vi "ServoSet.vi"(8 "error in":errorcluster, 10 "manual":dbl=0.03, 11 "Radio Buttons":T1(radio)) -> (0 "error out":errorcluster)   [LabVIEW 2016]
uses:
  <vilib>/DAQmx/create/channels.llb/DAQmx Create Channel (CO-Pulse Generation-Frequency).vi
  <vilib>/DAQmx/configure/timing.llb/DAQmx Timing (Implicit).vi
panel:
  in  "new duty cycle 2":dbl=0.5 min=0.001 max=0.999 step=0.001 format="%.6f"
  in  "idle state":i32(ring)=10214 items=["High"=10192, "Low"=10214]
  # "input roughly 0.008 ... 0.045"
  # "1\n24\n37\n48"
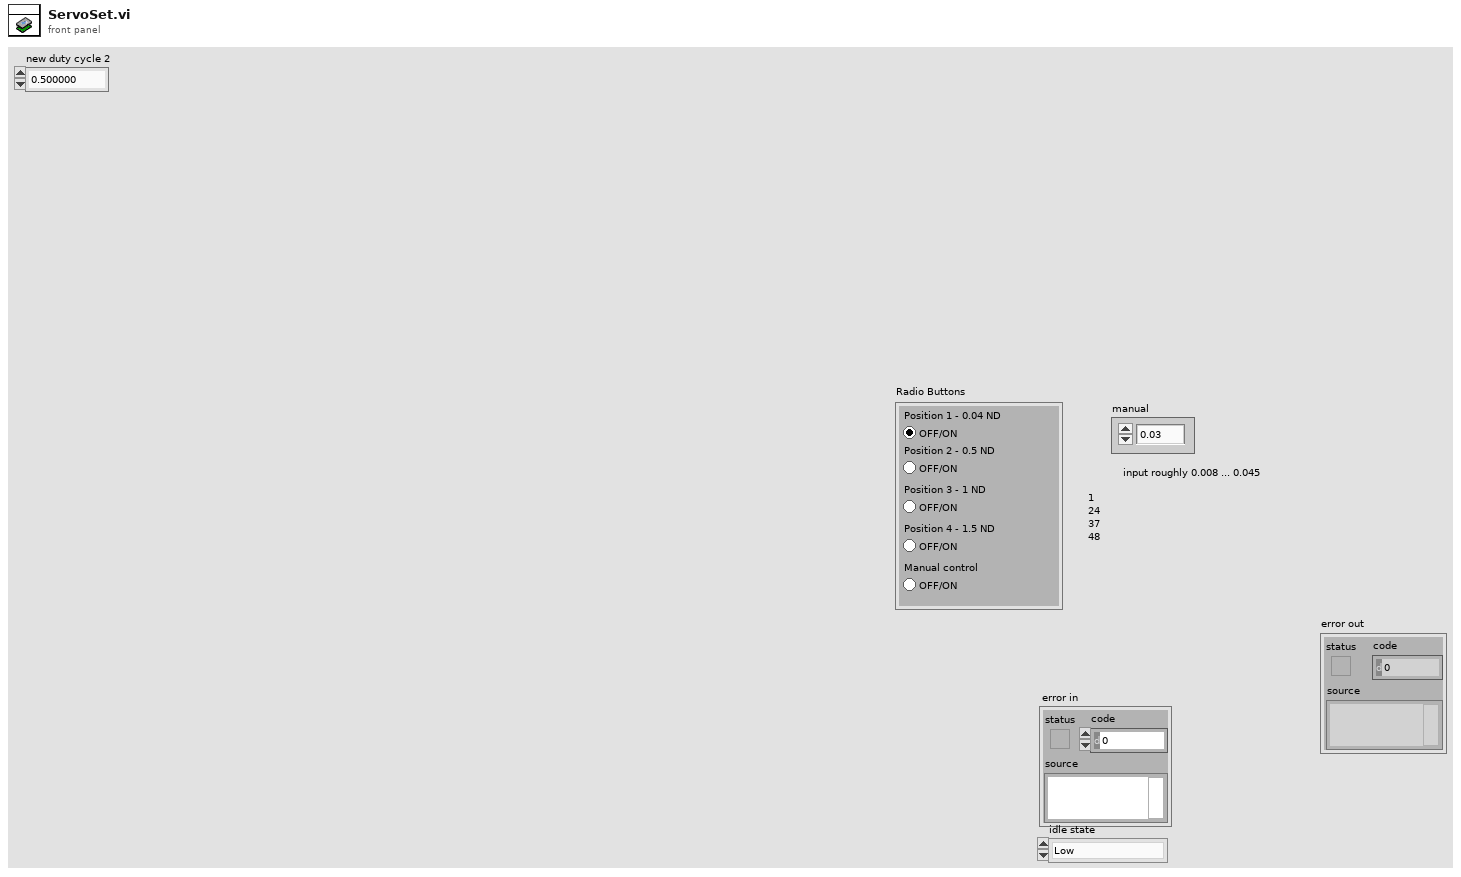
[diagram p1: front panel]
types:
  T1 = enum32{"Position 1 - 0.04 ND", "Position 2 - 0.5 ND", "Position 3 - 1 ND", "Position 4 - 1.5 ND", "Manual control"}
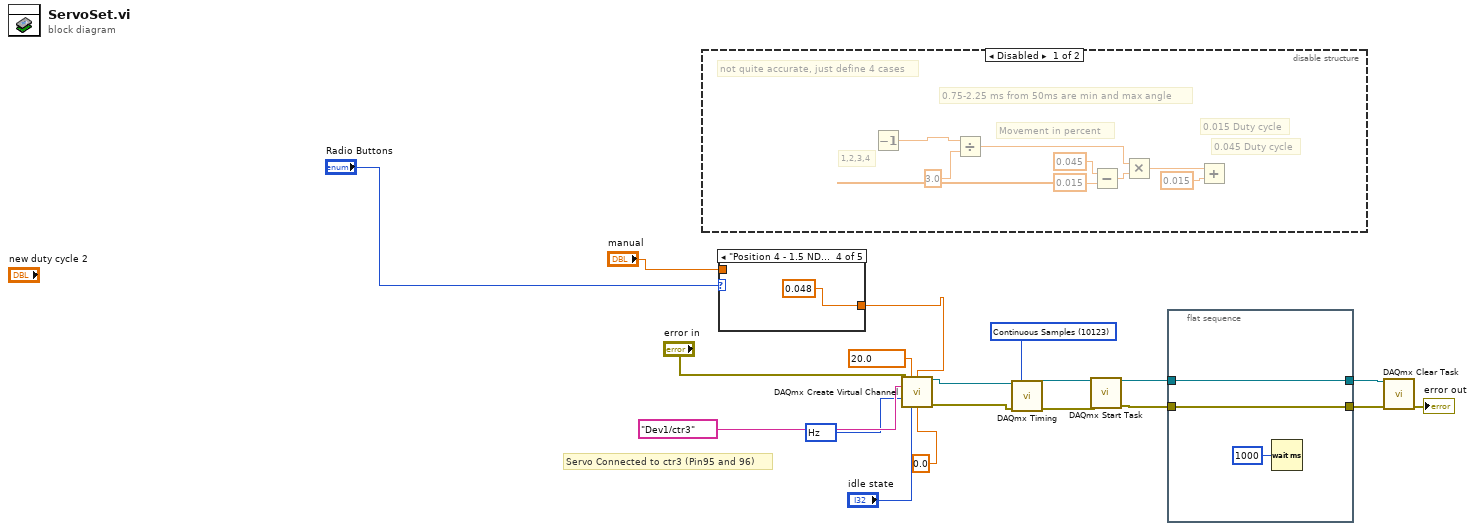
[diagram p0: block diagram]
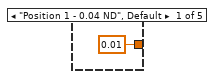
[diagram p2: hidden frame]
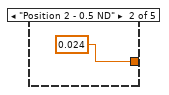
[diagram p3: hidden frame]
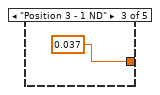
[diagram p4: hidden frame]
diagram:
  w14 = 10373 items=["Hz"=10373] ("units")
  w19 = 10123 items=["Finite Samples"=10178, "Continuous Samples"=10123, "Hardware Timed Single Point"=12522] ("sample mode")
  # "Servo Connected to ctr3 (Pin95 and 96)"
  n1 = disable-structure shown="Disabled" {
    frame Disabled {
      # "not quite accurate, just define 4 cases"
      # "1,2,3,4"
      # "0.015 Duty cycle"
      # "0.045 Duty cycle"
      # "0.75-2.25 ms from 50ms are min and max angle"
      # "Movement in percent"
      n2 = Decrement() -> (x=w21:dbl, x-1=w20:dbl)
      n3 = Divide(x=w20, y=3.0) -> (x/y=w23:dbl)
      n4 = Subtract(x=0.045, y=0.015) -> (x-y=w26:dbl)
      n5 = Multiply(x=w23, y=w26) -> (x*y=w25:dbl)
      n6 = Add(x=w25, y=0.015) -> ()  [unwired: 1 out]
    }
    frame Enabled {
    }
  }
  n7 = case shown="\"Position 4 - 1.5 ND\"" "Radio Buttons" {
    tunnel: [0.01 ("manual") 0.024 ("manual") 0.037 ("manual") 0.048 ("manual") w33] -> w4
    tunnel: "manual" -> [_ _ _ _ w33]
    frame "Position 1 - 0.04 ND", Default {
    }
    frame "Position 2 - 0.5 ND" {
    }
    frame "Position 3 - 1 ND" {
    }
    frame "Position 4 - 1.5 ND" {
    }
    frame "Manual control" {
    }
  }
  n8 = call-poly <vilib>:"DAQmx Create Virtual Channel.vi"("frequency"=20.0, "duty cycle"=w4, "counter"=tag "Dev1/ctr3" ("channel"), "units"=w14, "error in"="error in", "idle state"="idle state", "initial delay"=0.0) -> ("task out"=w18:refnum<k21>, "error out"=w10:errorcluster)  [unwired: 7 in]
  n9 = call-poly <vilib>:"DAQmx Timing.vi"("task/channels in"=w18, "sample mode"=w19, "error in"=w10) -> ("task out"=w16:refnum<k21>, "error out"=w9:errorcluster)  [unwired: 11 in]
  n10 = call <vilib>:"DAQmx Start Task.vi"("task/channels in"=w16, "error in"=w9) -> ("task out"=w7:refnum<k21>, "error out"=w6:errorcluster)  [unwired: 12 in]
  n11 = flat-sequence {
    tunnel: [w36] -> w8
    tunnel: w7 -> [w36]
    tunnel: w6 -> [w35]
    tunnel: [w35] -> w5
    frame #0 {
      n12 = Wait (ms)(milliseconds to wait=u32 1000) -> ()  [unwired: 1 out]
    }
  }
  n13 = call <vilib>:"DAQmx Clear Task.vi"("task in"=w8, "error in"=w5) -> ("error out"=→"error out":errorcluster)  [unwired: 13 in]
